vi "Init.vi"(8 "error in (no error)":errorcluster, 9 "Init Channels":T1[](array[typedef]), 11 "Info":T2) -> (0 "error out":errorcluster, 3 "Group out":refnum<class "Group.lvclass">)   [LabVIEW 2020, in "Vecto.lvlib" / "Group.lvclass"]
uses:
  Group.lvclass
  Group Info.ctl
  Channel Info.ctl
  Channel.ctl
  Channel Value.ctl
  Ref.ctl
  Group.lvclass/Group.ctl
  bf55b7b7-8edc-4f17-9daf-7d7c9d9b44fc.vi
  Vecto.lvlib
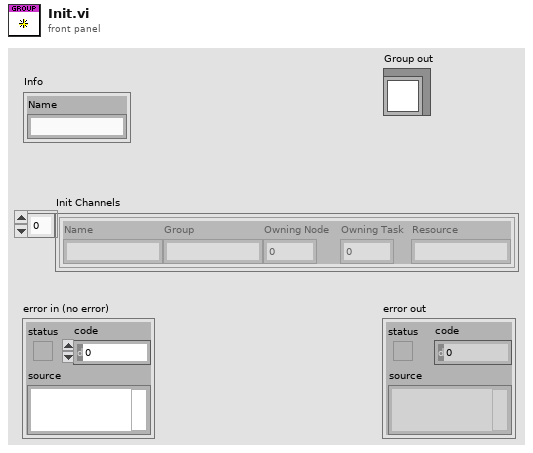
[diagram p1: front panel]
types:
  T1 = typedef "Vecto.lvlib/Channel Info.ctl" = cluster{"Name":string, "Group":string, "Owning Node":u32, "Owning Task":u32, "Resource":string}
  T2 = typedef "Vecto.lvlib/Group Info.ctl" = cluster{"Name":string}
  T3 = typedef "Vecto.lvlib/Channel.ctl" = cluster{"Info":T1, "Value":T4}
  T4 = typedef "Vecto.lvlib/Channel Value.ctl" = cluster{"Scaled":dbl, "Timestamp":dbl, "Raw":dbl}
  T5 = typedef "Vecto.lvlib/Group.lvclass/Ref.ctl" = cluster{"Channels":refnum<data-value>[], "Channel Index Map":map{string, i32}}
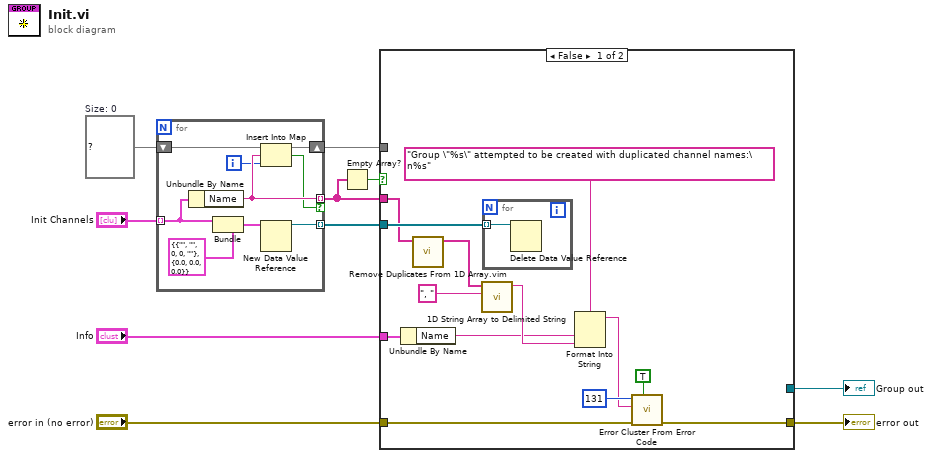
[diagram p0: block diagram]
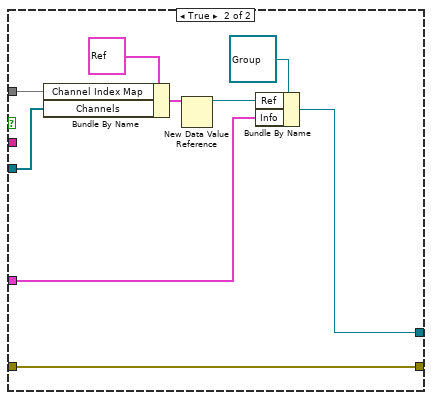
[diagram p2: hidden frame]
diagram:
  w7 = map{string, i32} {}  # Size: 0
  n1 = for {
    tunnel: "Init Channels" -> [w12] mode=indexing
    tunnel: [w19] -> w3 mode=indexing
    shift-right: [w17] -> w4
    shift-left: w7 -> [w18]
    tunnel: [w16] -> w2 mode=indexing if=w15
    i -> [w14]
    n2 = Unbundle By Name(w12) -> ("Name"=w16:string)
    n3 = Bundle(cluster=T3 {"Info"={"Name"="", "Group"="", "Owning Node"=0, "Owning Task"=0, "Resource"=""}, "Value"={"Scaled"=0.0, "Timestamp"=0.0, "Raw"=0.0}} ("Channel"), "Info"=w12) -> (w11:T3)  [unwired: 1 in]
    n4 = Insert Into Map(map in=w18, key=w16, value=w14) -> (map out=w17:map{string, i32}, key already included?=w15:bool)  [unwired: 1 out]
    n5 = New Data Value Reference(data value=w11) -> (data value reference=w19:refnum<data-value>)  [unwired: 1 in, 1 out]
  }
  n6 = Empty Array?(array=w2) -> (empty?=w1:bool)
  n7 = case shown="False" w1 {
    tunnel: [_ w41] -> w10
    tunnel: "Info" -> [w26 w39]
    tunnel: "error in (no error)" -> [w31 w38]
    tunnel: [w23 w38] -> w5
    tunnel: w4 -> [_ w36]
    tunnel: w3 -> [w32 w35]
    tunnel: w2 -> [w22 _]
    frame False {
      n8 = Unbundle By Name(w26) -> ("Name"=w20:string)
      n9 = call "Remove Duplicates From 1D Array.vim"("array"=w22) -> ("array with duplicates removed"=w21:string[])  [unwired: 10 in]
      n10 = call <vilib>:"1D String Array to Delimited String.vi"("delimiter"=", ", "string array"=w21) -> ("delimited string"=w25:string)  [unwired: 9 in]
      n11 = for {
        tunnel: w32 -> [w33] mode=indexing
        n12 = Delete Data Value Reference(data value reference=w33) -> ()  [unwired: 1 in, 2 out]
      }
      n13 = Format Into String(format string="Group \"%s\" attempted to be created with duplicated channel names:\n%s", w20, w25) -> (resulting string=w24:string)  [unwired: 2 in, 1 out]
      n14 = call <vilib>:"Error Cluster From Error Code.vi"("show call chain? (False)"=TRUE, "error in (no error)"=w31, "error message (\"\")"=w24, "error code (0)"=131) -> ("error out"=w23:errorcluster)  [unwired: 5 in]
    }
    frame True {
      n15 = Bundle By Name(cluster=T5 {"Channels"=[], "Channel Index Map"={}} ("Ref"), "Channel Index Map"=w36, "Channels"=w35) -> (w34:T5)
      n16 = New Data Value Reference(data value=w34) -> (data value reference=w40:refnum<data-value>)  [unwired: 1 in, 1 out]
      n17 = Bundle By Name(cluster=refnum<class "Group.lvclass"> refnum ("Group in"), "Ref"=w40, "Info"=w39) -> (w41:refnum<class "Group.lvclass">)
    }
  }
  "error out" <- w5
  "Group out" <- w10
